vi "Select Platform UI.vi"(8 "error in (no error)":errorcluster, 11 "Plugins":refnum<class "PlatformManager.lvclass">) -> (0 "error out":errorcluster, 2 "Cancelled":bool, 3 "Platform":string)   [LabVIEW 2020, in "PicoG-App.lvlib" / "picoG.lvclass"]
uses:
  picoG.lvclass
  Builds/picoG/ppl/PicoG-Core.lvlibp/PicoG-Processor/PicoG-Core/PlatformManager/PlatformManager.lvclass
panel:
  in  "Cancel":bool
  in  "OK":bool
  in  "Select Platform":string(combo)
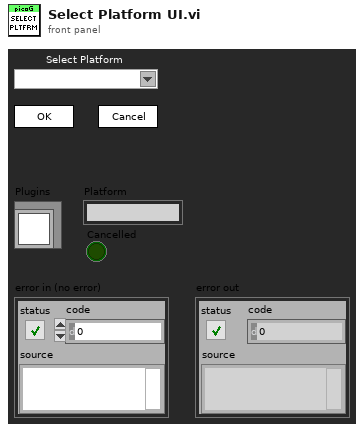
[diagram p1: front panel]
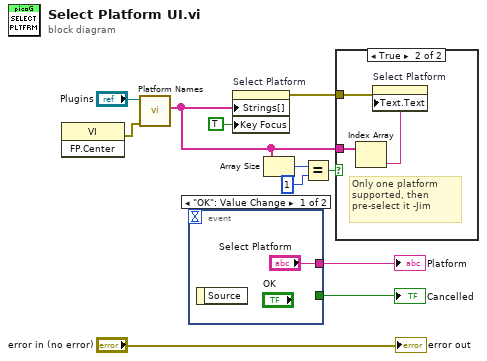
[diagram p0: block diagram]
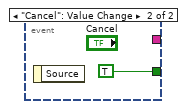
[diagram p3: hidden frame]
diagram:
  n1 = invoke class="VI" method="FP.Center"() -> (error out=w1:errorcluster)  [unwired: 3 in, 2 out]
  n2 = call "Platform Names.vi"("error in (no error)"=w1, "PlatformManager in"="Plugins") -> ("Platforms"=w4:string[])  [unwired: 7 in, 2 out]
  n3 = event shown="[0] \"OK\": Value Change" {
    selector: _ -> [_ _]
    dyn-events: _ -> [_ _]
    timeout: _ -> [_ _]
    tunnel: ["Select Platform" _] -> w10
    tunnel: [_ TRUE] -> w9
    event "OK": Value Change {
      n4 = event-data() -> ()  [unwired: 1 in, 1 out]
    }
    event "Cancel": Value Change {
      n5 = event-data() -> ()  [unwired: 1 in, 1 out]
    }
  }
  "Platform" <- w10
  "Cancelled" <- w9
  n6 = property on="Select Platform" class="CmbBox"("Strings[]"=w4, "Key Focus"=TRUE) -> (error out=w5:errorcluster)  [unwired: 2 in, 1 out]
  n7 = Array Size(array=w4) -> (size(s)=w8:i32)
  n8 = Equal?(x=w8, y=1) -> (x = y?=w6:bool)
  n9 = case shown="True" w6 {
    tunnel: w5 -> [_ w16]
    tunnel: w4 -> [_ w15]
    frame False {
    }
    frame True {
      # "Only one platform supported, then pre-select it -Jim"
      n10 = Index Array(array=w15) -> (element=w14:string)  [unwired: 1 in]
      n11 = property on="Select Platform" class="CmbBox"(error in=w16, "Text.Text"=w14) -> ()  [unwired: 1 in, 2 out]
    }
  }
  "error out" <- "error in (no error)"
